vi "Sector Parameter Global.vi"() -> ()   [LabVIEW 2013]
uses:
  Sector/Accumulate/Sector Parameter Cluster.ctl
panel:
  out "Left + Right Cycle Output":fxp<+,8,0>
  in  "Preanalysis Right Sector":u8
  in  "Preanalysis Left Sector":u8
  in  "Right Analysis End Angle":fxp<+/-,17,2>
  in  "Right Analysis Start Angle":fxp<+/-,17,2> caption="2nd Analysis Start Angle (PI Radians)"
  in  "Left Analysis End Angle":fxp<+/-,17,2>
  in  "Left Analysis Start Angle":fxp<+/-,17,2> caption="2nd Analysis Start Angle (PI Radians)"
  out "Left - Right Cycle Output":fxp<+,8,0>
  out "Right Duty Cycle Output":fxp<+/-,9,1>
  out "Left Duty Cycle Output":fxp<+/-,9,1>
  in  "Right Start Angle Duty Cycle":fxp<+,8,0>
  in  "Right End Angle Duty Cycle":fxp<+,8,0>
  in  "Left End Angle Duty Cycle":fxp<+,8,0>
  in  "Left Start Angle Duty Cycle":fxp<+,8,0>
  in  "Sector Threshold":u8
  in  "[Average BG Intensity]":u8[](array[numeric])=[0, 0, 0, 0, 0, 0, 0, 0, 0, 0, 0, 0, 0, 0, 0, 0, 0, 0, 0, 0, 0, 0, 0, 0, 0, 0, 0, 0, 0, 0, 0, 0]
  in  "Sector Parameters Right":T1
  in  "Sector Parameters Left":T1={"Start Angle"=0.65740966796875, "End Angle"=0.99468994140625, "Inner Radius"=309, "Outter Radius"=405, "Hinge X"=464, "Hinge Y"=534, "NumWingSectors"=8}
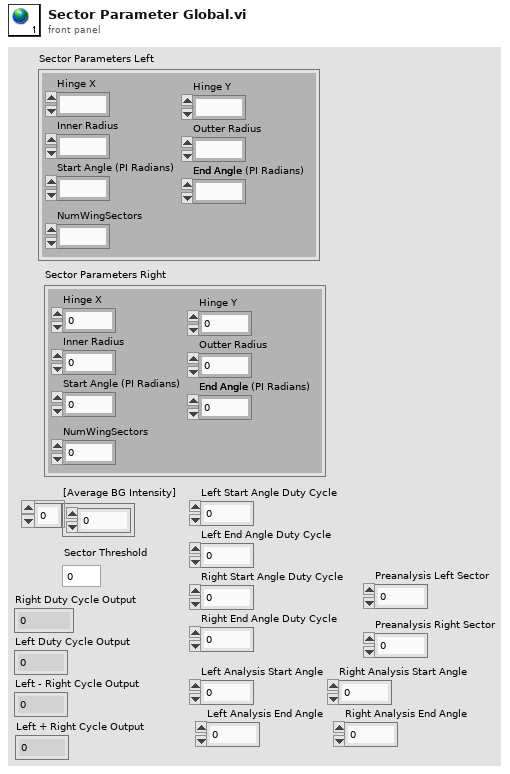
[diagram p1: front panel]
types:
  T1 = typedef "Sector Parameter Cluster.ctl" = cluster{"Start Angle":fxp<+/-,17,2>, "End Angle":fxp<+/-,17,2>, "Inner Radius":u16, "Outter Radius":u16, "Hinge X":u16, "Hinge Y":u16, "NumWingSectors":u8}
diagram:
